vi "user output.vi"(8 "error in":errorcluster, 11 "Outputs to system":T1) -> (0 "error out":errorcluster)   [LabVIEW 2013, in "user control module.lvclass"]
uses:
  user control module.lvclass
  output user data.ctl
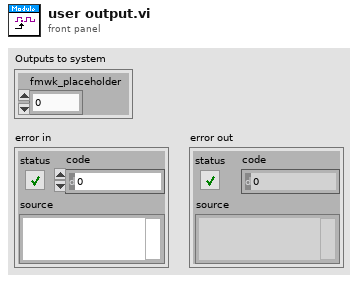
[diagram p1: front panel]
types:
  T1 = typedef "user control module.lvclass/output user data.ctl" = cluster{"fmwk_placeholder":sgl}
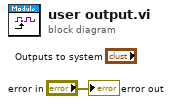
[diagram p0: block diagram]
diagram:
  "error out" <- "error in"
